vi "get_focus_edges.vi"(6 "Focus function":enum16{"Std dev", "Edges std dev"}(ring)=enum."Edges std dev", 8 "error in (no error)":errorcluster, 10 "Mask out":T1, 11 "Image in":T1) -> (0 "error out":errorcluster, 3 "Global Report":T2)   [LabVIEW 2011]
uses:
  <vilib>/vision/Image Controls.llb/IMAQ Image.ctl
  <vilib>/vision/NI_Vision_Development_Module.lvlib
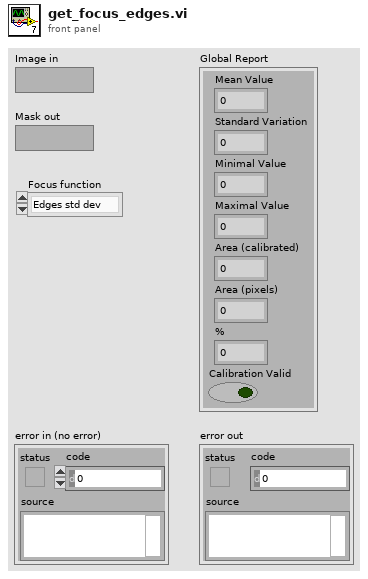
[diagram p1: front panel]
types:
  T1 = typedef "IMAQ Image.ctl" = refnum<image>
  T2 = cluster{"Mean Value":sgl, "Standard Variation":sgl, "Minimal Value":sgl, "Maximal Value":sgl, "Area (calibrated)":sgl, "Area (pixels)":u32, "%":sgl, "Calibration Valid":bool}
  T3 = enum32{"Differentiation", "Gradient", "Prewitt", "Roberts", "Sigma", "Sobel"}
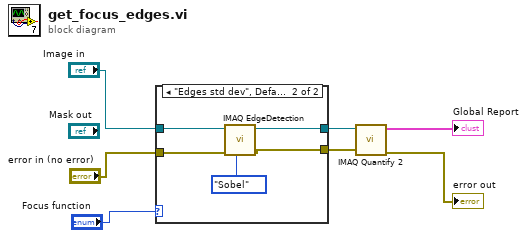
[diagram p0: block diagram]
diagram:
  n1 = case shown="\"Edges std dev\", Default" "Focus function" {
    tunnel: "Image in" -> [w9 w14]
    tunnel: "error in (no error)" -> [w8 w13]
    tunnel: [w9 w12] -> w3
    tunnel: [w8 w11] -> w2
    frame "Std dev" {
    }
    frame "Edges std dev", Default {
      n2 = call "IMAQ EdgeDetection"("Method"=T3."Sobel", "error in (no error)"=w13, "Image Src"=w14) -> ("error out"=w11:errorcluster, "Image Dst Out"=w12:T1)  [unwired: 7 in]
    }
  }
  n3 = call "IMAQ Quantify 2"("error in (no error)"=w2, "Image"=w3) -> ("error out"=→"error out":errorcluster, "Global Report"=→"Global Report":T2)  [unwired: 7 in, 1 out]
